vi "caller.vi"(0 "TDMS File Path":path, 5 "Stop":bool, 11 "Error In":errorcluster) -> (15 "Error Out":errorcluster)   [LabVIEW 2023]
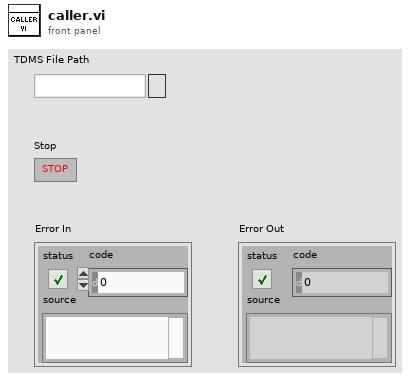
[diagram p1: front panel]
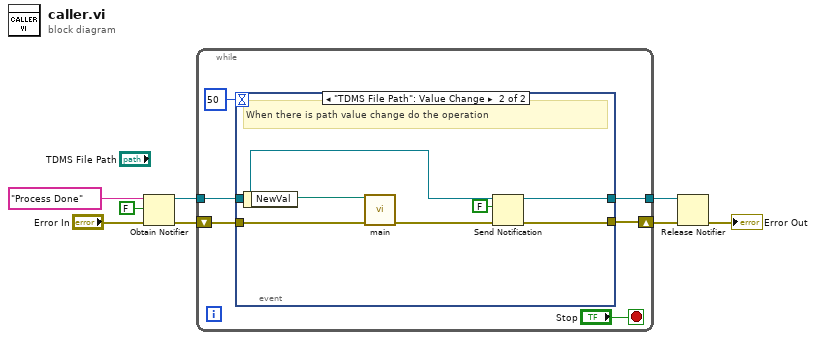
[diagram p0: block diagram]
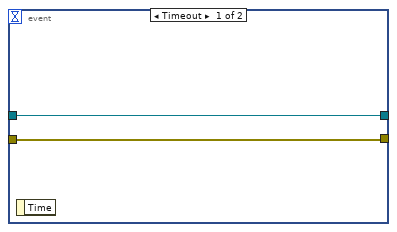
[diagram p2: hidden frame]
diagram:
  n1 = Obtain Notifier(name (unnamed)="Process Done", notification data type=FALSE, error in (no error)="Error In") -> (notifier out=w3:refnum<notifier>, error out=w6:errorcluster)  [unwired: 1 in, 1 out]
  n2 = while {
    shift-right: [w12] -> w7
    shift-left: w6 -> [w13]
    tunnel: w3 -> [w10]
    tunnel: [w9] -> w1
    stop <- "Stop" stop-if-true
    n3 = event shown="[1] \"TDMS File Path\": Value Change" {
      selector: _ -> [_ _]
      dyn-events: _ -> [_ _]
      timeout: 50 -> [_ _]
      tunnel: [w16 w20] -> w12
      tunnel: w13 -> [w16 w23]
      tunnel: [w15 w18] -> w9
      tunnel: w10 -> [w15 w19]
      event Timeout {
        n4 = event-data() -> ()  [unwired: 1 in, 1 out]
      }
      event "TDMS File Path": Value Change {
        # "When there is path value change do the operation"
        n5 = event-data() -> ("NewVal"=w21:path)  [unwired: 1 in]
        n6 = call "main.vi"("TDMS File Path"=w21, "Error In"=w23) -> ("Error Out"=w22:errorcluster)  [unwired: 13 in]
        n7 = Send Notification(notification=FALSE, notifier=w19, error in (no error)=w22) -> (notifier out=w18:refnum<notifier>, error out=w20:errorcluster)
      }
    }
  }
  n8 = Release Notifier(notifier=w1, error in (no error)=w7) -> (error out=→"Error Out":errorcluster)  [unwired: 1 in, 2 out]
